vi "Not Equal Float.vi"(1 "Comparison \nTolerance":dbl=0.001 format="%.4f", 2 "Input 2":dbl format="%.2f", 3 "Input 1":dbl format="%.2f") -> (0 "Not Equal":bool)   [LabVIEW 2016]
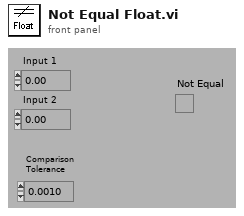
[diagram p1: front panel]
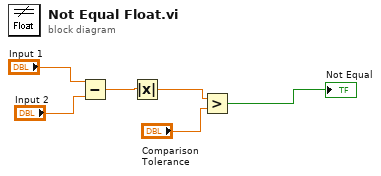
[diagram p0: block diagram]
diagram:
  n1 = Subtract(x="Input 1", y="Input 2") -> (x-y=w4:dbl)
  n2 = Absolute Value(x=w4) -> (abs(x)=w3:dbl)
  n3 = Greater?(x=w3, y="Comparison \nTolerance") -> (0:→"Not Equal":bool)
